vi "Execute InrTerm Handle.vi"(6 "Menu Item Tag Suffix":string, 8 "错误输入（无错误）":errorcluster, 11 "内部接线端输入":refnum<vi>) -> (0 "错误输出":errorcluster)   [LabVIEW 2020]
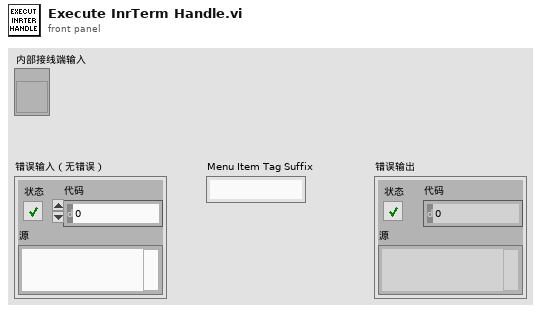
[diagram p1: front panel]
types:
  T1 = typedef "LVRectTypeDef.ctl" = cluster{"Left":i16, "Top":i16, "Right":i16, "Bottom":i16}
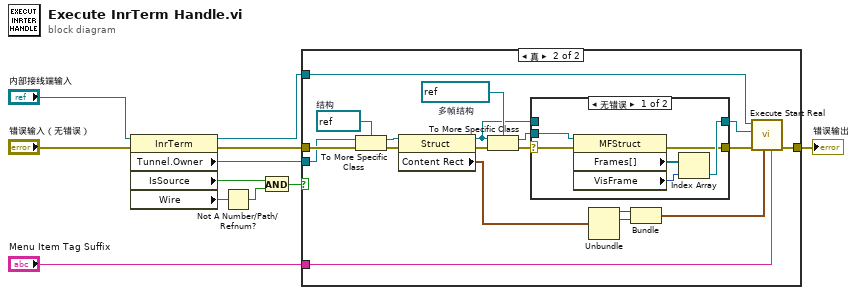
[diagram p0: block diagram]
diagram:
  n1 = property class="InrTerm"(reference="内部接线端输入", error in="错误输入（无错误）") -> (reference out=w9:refnum<vi>, error out=w8:errorcluster, "Tunnel.Owner"=w11:refnum<vi>, "IsSource"=w7:bool, "Wire"=w1:refnum<vi>)
  n2 = Not A Number/Path/Refnum?(number/path/refnum=w1) -> (NaN/Path/Refnum?=w2:bool)
  n3 = And(x=w7, y=w2) -> (x .and. y?=w3:bool)
  n4 = case shown="真" w3 {
    tunnel: w8 -> [w12 w31]
    tunnel: w9 -> [_ w16]
    tunnel: "Menu Item Tag Suffix" -> [_ w13]
    tunnel: w11 -> [_ w25]
    tunnel: [w12 w14] -> w4
    frame False {
    }
    frame True {
      w23 = refnum<vi> refnum  # 结构
      w30 = refnum<vi> refnum  # 多帧结构
      n5 = To More Specific Class(target class=w23, reference=w25, error in=w31) -> (specific class reference=w24:refnum<vi>, error out=w26:errorcluster)
      n6 = property class="Struct"(reference=w24, error in=w26) -> (reference out=w17:refnum<vi>, error out=w27:errorcluster, "Content Rect"=w19:T1)
      n7 = To More Specific Class(target class=w30, reference=w17, error in=w27) -> (specific class reference=w29:refnum<vi>, error out=w28:errorcluster)
      n8 = case shown="无错误" w28 {
        selector: w28 -> [w34 _]
        tunnel: w29 -> [w37 _]
        tunnel: [w33 w38] -> w18
        tunnel: w17 -> [_ w38]
        tunnel: [w32 _] -> w15
        frame No Error {
          n9 = property class="MFStruct"(reference=w37, error in=w34) -> (error out=w32:errorcluster, "Frames[]"=w36:refnum<vi>[], "VisFrame"=w35:u32)  [unwired: 1 out]
          n10 = Index Array(array=w36, index=w35) -> (element=w33:refnum<vi>)
        }
        frame Error {
        }
      }
      n11 = Unbundle(w19) -> ("Left"=w22:i16, "Top"=w21:i16)  [unwired: 2 out]
      n12 = Bundle("Left"=w22, "Top"=w21) -> (w20:cluster{"Left":i16, "Top":i16})  [unwired: 1 in]
      n13 = call "Execute Start Real.vi"("Menu Item Tag Suffix"=w13, "相对位置原点"=w20, "错误输入（无错误）"=w15, "所有者引用句柄"=w18, "接线端输入"=w16) -> ("错误输出"=w14:errorcluster)  [unwired: 6 in]
    }
  }
  "错误输出" <- w4
